vi "Pop.vi"(8 "Error In":errorcluster, 11 "Context In":refnum<class "Context.lvclass">) -> (0 "Error Out":errorcluster, 2 "Datum":refnum<class "Abstract.lvclass">, 3 "Context Out":refnum<class "Context.lvclass">)   [LabVIEW 2018, in "Toolkit.lvlib" / "Data.lvlib" / "Context.lvclass"]
uses:
  Context.lvclass
  Abstract/Abstract.lvclass
  Context.lvclass/Context.ctl
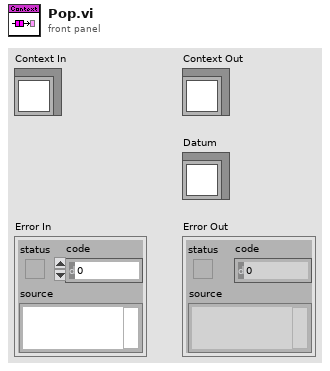
[diagram p1: front panel]
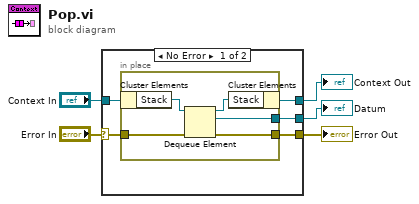
[diagram p0: block diagram]
diagram:
  n1 = case shown="No Error" "Error In" {
    selector: "Error In" -> [w8 w16]
    tunnel: [w7 w16] -> w4
    tunnel: [w9 w17] -> w2
    tunnel: "Context In" -> [w10 w17]
    tunnel: [w6 _] -> w1
    frame No Error {
      n2 = in-place {
        in-place-border: w8 -> [w13]
        in-place-border: [w12] -> w7
        in-place-border: [w11] -> w6
        n3 = in-place-cluster #1(w10) -> ("Stack"=w15:refnum<queue>)
        n4 = Dequeue Element(queue=w15, error in (no error)=w13) -> (queue out=w14:refnum<queue>, element=w11:refnum<class "Abstract.lvclass">, error out=w12:errorcluster)  [unwired: 1 in, 1 out]
        n5 = in-place-cluster #1("Stack"=w14) -> (w9:refnum<class "Context.lvclass">)
      }
    }
    frame Error {
    }
  }
  "Error Out" <- w4
  "Context Out" <- w2
  "Datum" <- w1
